vi "test.vi"() -> ()   [LabVIEW 2017]
uses:
  Resource Agents/Development/Battery/2017.12 - BA v0.5/General purpose/daemon-config.ctl
panel:
  out "JSON string":string
  in  "daemon-config":T1={"resource-type"="battery", "agent-id"=12, "GA-ip"="192.168.1.1", "GA-port"=52020, "RA-ip"="127.0.0.1", "RA-port"=52001, "listenport-RA-side"=52011, "listenport-GA-side"=52021, "local-ip"="192.168.1.12", "long-term"=FALSE}
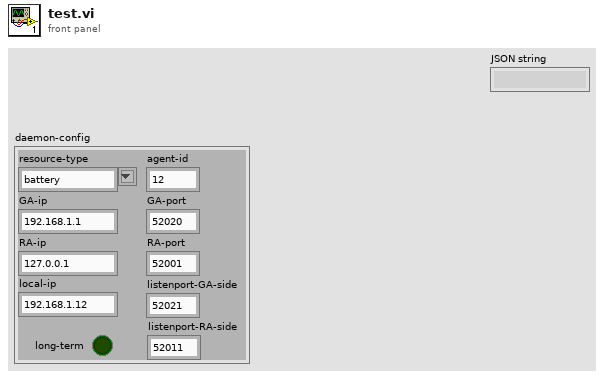
[diagram p1: front panel]
types:
  T1 = typedef "daemon-config.ctl" = cluster{"resource-type":string, "agent-id":u16, "GA-ip":string, "GA-port":u16, "RA-ip":string, "RA-port":u16, "listenport-RA-side":u16, "listenport-GA-side":u16, "local-ip":string, "long-term":bool}
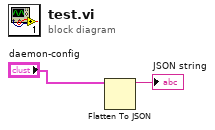
[diagram p0: block diagram]
diagram:
  n1 = Flatten To JSON(anything="daemon-config") -> (JSON string=→"JSON string":string)  [unwired: 2 in, 1 out]
